vi "Field Centric Test.vi"() -> ()   [LabVIEW 2020]
panel:
  out "Arcade Inputs":picture
  out "XY Graph":cluster{dbl[], dbl[]}[](graph)
  in  "IMU":dbl(slide) scale=-180.0..180.0
  # "Front (-1)"
  # "Left (-1)"
  # "Right (1)"
  # "Back (1)"
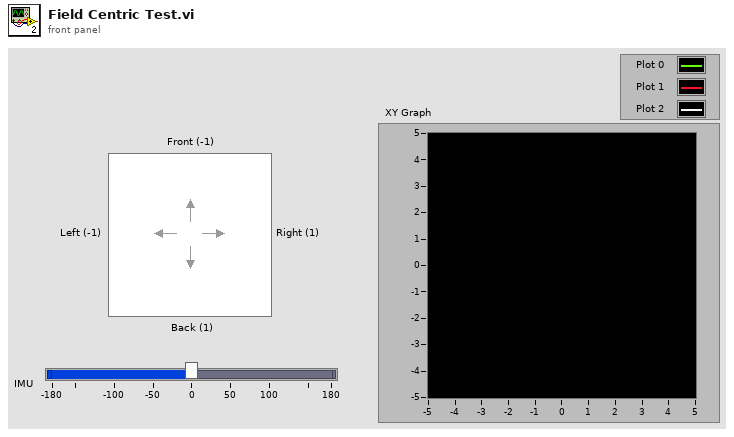
[diagram p1: front panel]
types:
  T1 = typedef "LVMouseTypeDef.ctl" = cluster{"Mouse Position":cluster{"X":i32, "Y":i32}, "Mouse Modifiers":cluster{"Button Down":bool, "Shift Mod":bool, "Menu Mod":bool, "Option Mod":bool}}
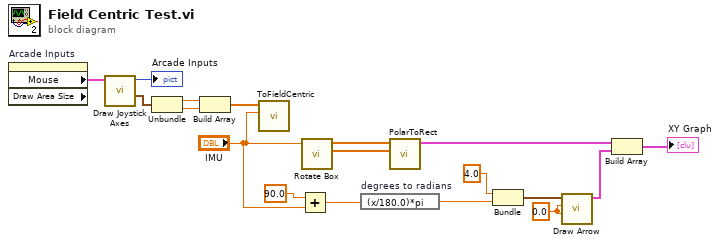
[diagram p0: block diagram]
diagram:
  w12 = 0.0 ("Start X")
  n1 = property on="Arcade Inputs" class="Pict" props=["Mouse", "Draw Area Size"]() -> ("Mouse"=w15:T1)  [unwired: 2 in, 3 out]
  n2 = call "Draw Joystick Axes.vi"("Mouse"=w15) -> ("JS Coords"=w14:cluster{"X":dbl, "Y":dbl}, "Arcade Inputs"=→"Arcade Inputs":picture)  [unwired: 9 in]
  n3 = Unbundle(w14) -> ("X"=w18:dbl, "Y"=w17:dbl)
  n4 = Build Array(w18, w17) -> (w13:dbl[])
  n5 = call "ToFieldCentric.vi"("IMU Value (offset)"="IMU", "Vectors"=w13) -> ()  [unwired: 9 in, 1 out]
  n6 = Add(x=90.0, y="IMU") -> (x+y=w1:dbl)
  n7 = call "Rotate Box.vi"("IMU"="IMU") -> ("theta"=w11:dbl[], "r"=w9:dbl[])  [unwired: 7 in]
  n8 = expression code="(x/180.0)*pi" "degrees to radians"(w1) -> (w10:dbl)
  n9 = call "PolarToRect.vi"("theta"=w11, "r"=w9) -> ("Rectangular Coordinates"=w5:cluster{dbl[], dbl[]})  [unwired: 9 in]
  n10 = Bundle("Start X"=4.0, w10) -> (w7:cluster{"Start X":dbl, dbl})  [unwired: 1 in]
  n11 = call "Draw Arrow.vi"("Start Y"=w12, "Start X"=w12, "Pod Setpoint"=w7) -> ("Points"=w6:cluster{dbl[], dbl[]})  [unwired: 6 in, 2 out]
  n12 = Build Array(w5, w6) -> (→"XY Graph":cluster{dbl[], dbl[]}[])
